vi "Main.vi"() -> ()   [LabVIEW 2017]
doc: "The myRIO Project template acquires acceleration data from the onboard accelerometer and displays the changes of acceleration values in a waveform chart."
uses:
  Projekt-RubikLibrary/ServoEnumControl.ctl
  Projekt-RubikLibrary/ServoAbsAngleControl.ctl
  <vilib>/myRIO/Common/Instrument Driver Framework/myRIO v1.0/UART/vis/myRIO v1.0 Close UART.vi
  <vilib>/myRIO/Common/Instrument Driver Framework/Utilities/vis/FPGA Ref Manager.vi
  <vilib>/myRIO/Common/Instrument Driver Framework/myRIO v1.0/myRIO v1.0 Reset FPGA.vi
  <vilib>/myRIO/Common/Instrument Driver Framework/myRIO v1.0/IRQ/vis/myRIO v1.0 IRQ Info FGV.vi
  <vilib>/myRIO/Common/Instrument Driver Framework/myRIO v1.0/IRQ/vis/myRIO v1.0 Timer IRQ Info FGV.vi
  <vilib>/myRIO/Common/Instrument Driver Framework/myRIO v1.0/IRQ/vis/myRIO v1.0 ISR Agent.vi
  <vilib>/ErrorRing/Error Ring.xnode
  <vilib>/myRIO/Instrument Drivers/Utilities/Utilities.lvlib
  Projekt-RubikLibrary/RubikLibrary.lvlib
panel:
  out "error out":errorcluster
  in  "Stop":bool
  # "Test Orientation Finite State Machine of Rubik's Cube"
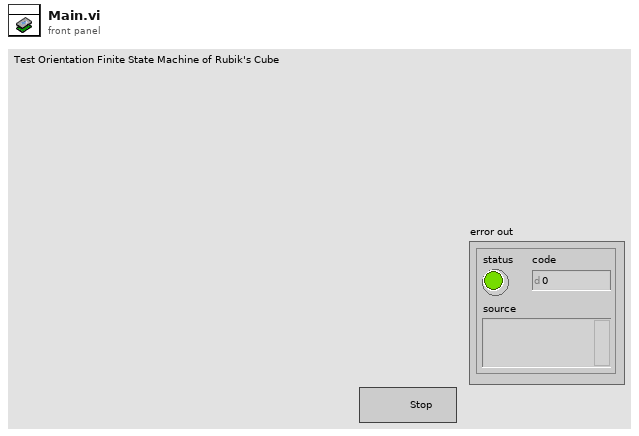
[diagram p1: front panel]
types:
  T1 = typedef "RubikLibrary.lvlib/ServoAbsAngleControl.ctl" = enum16{"+90°", "0°", "-90°"}
  T2 = typedef "RubikLibrary.lvlib/ServoEnumControl.ctl" = enum16{"Left Servo", "Front Servo", "Right Servo"}
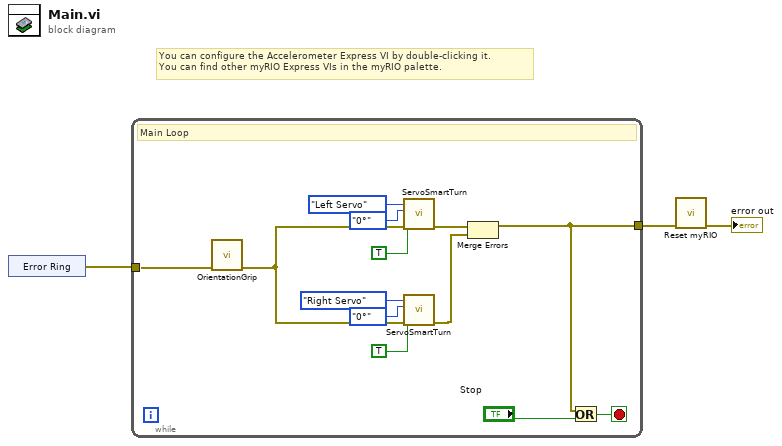
[diagram p0: block diagram]
diagram:
  # "You can configure the Accelerometer Express VI by double-clicking it.\nYou can find other myRIO Express VIs in the myRIO palette."
  n1 = xnode "Error Ring"() -> ("error out"=w1:errorcluster)
  n2 = while {
    tunnel: w1 -> [w5]
    tunnel: [w11] -> w3
    stop <- w15 stop-if-true
    # "Main Loop"
    n3 = call "OrientationGrip.vi"("error in"=w5) -> ("error out"=w4:errorcluster)  [unwired: 10 in]
    n4 = call "ServoSmartTurn.vi"("error in"=w4, "NoWait"=TRUE, "Turn to (in)"=ServoAbsAngleControl."0°", "Servo"=ServoEnumControl."Left Servo") -> ("error out"=w12:errorcluster)  [unwired: 6 in, 1 out]
    n5 = call "ServoSmartTurn.vi"("error in"=w4, "NoWait"=TRUE, "Turn to (in)"=ServoAbsAngleControl."0°", "Servo"=ServoEnumControl."Right Servo") -> ("error out"=w10:errorcluster)  [unwired: 6 in, 1 out]
    n6 = Merge Errors(w12, w10) -> (w11:errorcluster)
    n7 = Or(x=w11, y="Stop") -> (x .or. y?=w15:bool)
  }
  n8 = call <vilib>:"Reset myRIO.vi"("error in (no error)"=w3) -> ("error out"=→"error out":errorcluster)  [unwired: 10 in]
